vi "Lock.vi"(8 "error out":errorcluster, 11 "VISA resource name":refnum<visa-resource-name>) -> (0 "error out":errorcluster, 2 "locked?":bool, 3 "VISA resource name out":refnum<visa-resource-name>, 4 "Device Errors":cluster{"code":i32, "Text":string}[](array[cluster]))   [LabVIEW 2014, in "Stanford Research DG645 - Driver.lvlib"]
doc: "Interface Command: LOCK?\nInstrument Error Check\n\nRequest the instrument lock. The DG645 returns true if the lock is granted and false otherwise. When the lock is granted, no other instrument interface may alter instrument settings until the lock has released via the UNLK command."
uses:
  Stanford Research DG645 - Driver.lvlib
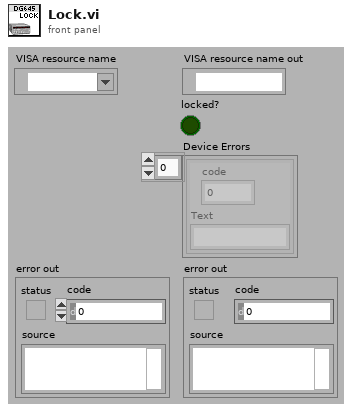
[diagram p1: front panel]
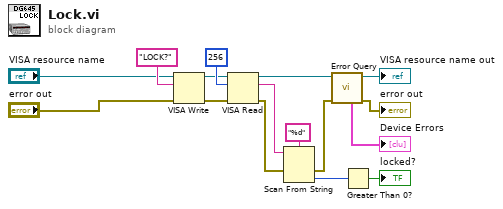
[diagram p0: block diagram]
diagram:
  n1 = VISA Write(VISA resource name="VISA resource name", write buffer="LOCK?" ("ID Query"), error in (no error)="error out") -> (VISA resource name out=w9:refnum<visa-resource-name>, error out=w7:errorcluster)  [unwired: 1 out]
  n2 = VISA Read(VISA resource name=w9, byte count=u32 256, error in (no error)=w7) -> (VISA resource name out=w8:refnum<visa-resource-name>, read buffer=w2:string, error out=w4:errorcluster)  [unwired: 1 out]
  n3 = Scan From String(format string="%d", input string=w2, error in=w4) -> (error out=w3:errorcluster, output 1=w5:i32)  [unwired: 2 in, 2 out]
  n4 = call "Error Query.vi"("error in (no error)"=w3, "VISA resource name"=w8) -> ("error out"=→"error out":errorcluster, "VISA resource name out"=→"VISA resource name out":refnum<visa-resource-name>, "Device Errors"=→"Device Errors":cluster{"code":i32, "Text":string}[])  [unwired: 7 in]
  n5 = Greater Than 0?(x=w5) -> (x > 0?=→"locked?":bool)
